vi "ReadBOTUpdates.vi"(0 "reference in":refnum<class "TelegramBOT.lvclass">, 5 "error in (no error)":errorcluster) -> (14 "reference out":refnum<class "TelegramBOT.lvclass">, 16 "result":T1[](array[typedef]), 17 "Connection":bool, 19 "error out":errorcluster)   [LabVIEW 2014, in "TelegramBOT.lvclass"]
uses:
  TelegramBOT.lvclass
  UpdateResultElem.ctl
  QueryStringElem.ctl
  <vilib>/httpClient/LabVIEWHTTPClient.lvlib
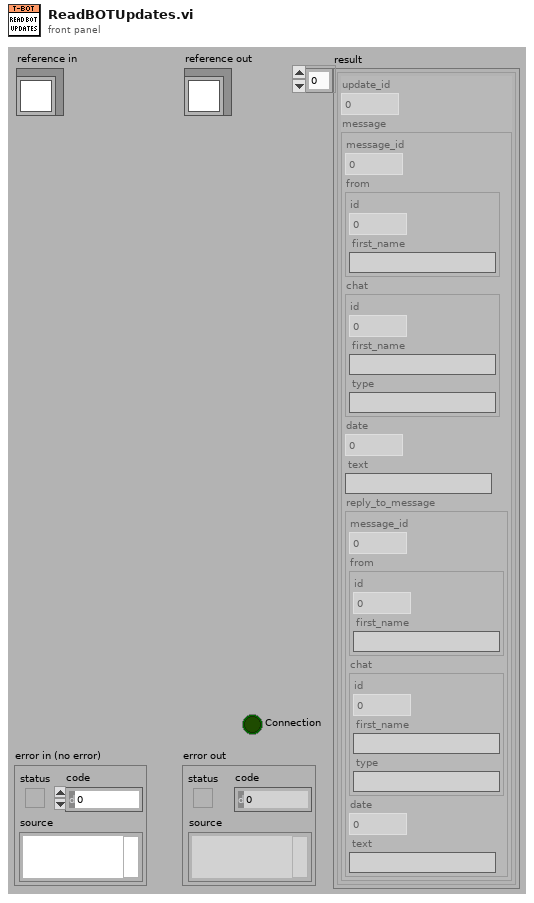
[diagram p1: front panel]
types:
  T1 = typedef "TelegramBOT.lvclass/UpdateResultElem.ctl" = cluster{"update_id":u32, "message":cluster{"message_id":u32, "from":cluster{"id":u64, "first_name":string}, "chat":cluster{"id":i32, "first_name":string, "type":string}, "date":u32, "text":string, "reply_to_message":cluster{"message_id":u32, "from":cluster{"id":u64, "first_name":string}, "chat":cluster{"id":i32, "first_name":string, "type":string}, "date":u32, "text":string}}}
  T2 = typedef "TelegramBOT.lvclass/QueryStringElem.ctl" = cluster{"QueryString":string, "QueryStringValue":string}
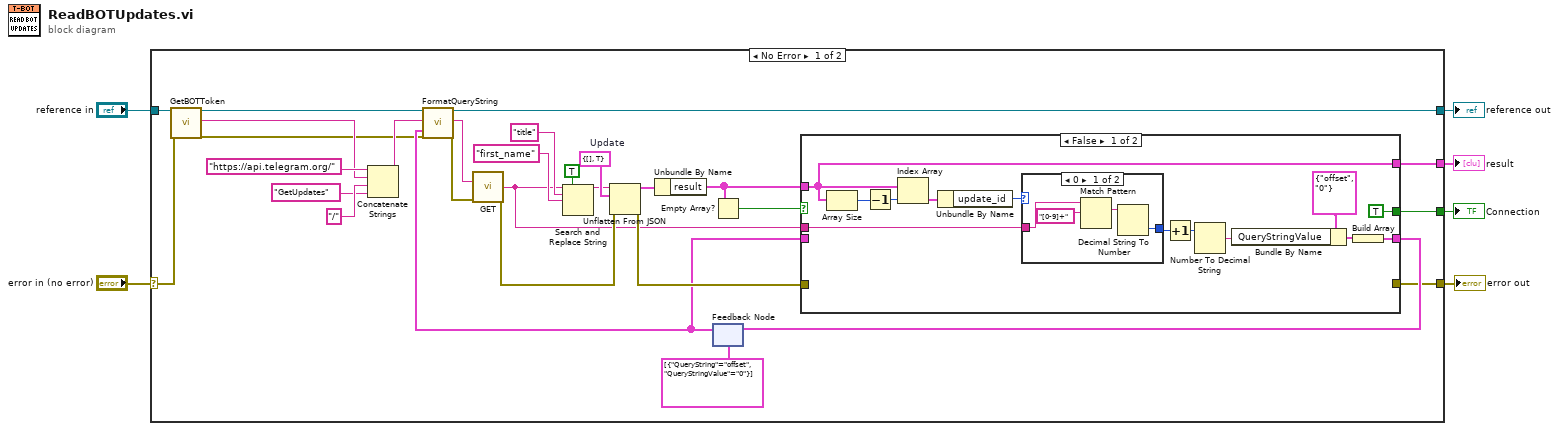
[diagram p0: block diagram]
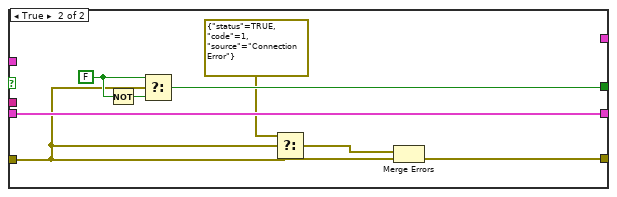
[diagram p3: hidden frame]
diagram:
  n1 = case shown="No Error" "error in (no error)" {
    selector: "error in (no error)" -> [w34 w63]
    tunnel: [w10 w63] -> w5
    tunnel: [w13 w62] -> w3
    tunnel: "reference in" -> [w35 w62]
    tunnel: [w8 _] -> w2
    tunnel: [w7 _] -> w1
    frame No Error {
      w32 = cluster{"result":T1[], "ok":bool} {"result"=[], "ok"=TRUE}  # Update
      n2 = call "GetBOTToken.vi"("reference in"=w35, "error in (no error)"=w34) -> ("reference out"=w14:refnum<class "TelegramBOT.lvclass">, "BOTToken"=w19:string, "error out"=w12:errorcluster)  [unwired: 15 in]
      n3 = Concatenate Strings("https://api.telegram.org/" ("URL"), w19, "/" ("URL"), "GetUpdates" ("URL")) -> (w17:string)
      n4 = feedback #1(T2[] [{"QueryString"="offset", "QueryStringValue"="0"}] ("QueryStringItems")) -> (w15:T2[])
      n5 = call "FormatQueryString.vi"("reference in"=w14, "QueryStringIn"=w17, "QueryStringItems"=w15, "error in (no error)"=w12) -> ("reference out"=w13:refnum<class "TelegramBOT.lvclass">, "QueryStringOut"=w16:string, "error out"=w11:errorcluster)  [unwired: 13 in]
      n6 = call <vilib>:"GET.vi"("url"=w16, "error in (no error)"=w11) -> ("body"=w21:string, "error out"=w27:errorcluster)  [unwired: 10 in, 2 out]
      n7 = Search and Replace String(replace all?=TRUE ("replace all? (F)"), input string=w21, search string="title" ("input string"), replace string="first_name" ("input string")) -> (result string=w28:string)  [unwired: 4 in, 3 out]
      n8 = Unflatten From JSON(JSON string=w28, type and defaults=w32, error in (no error)=w27) -> (value=w24:cluster{"result":T1[], "ok":bool}, error out=w26:errorcluster)  [unwired: 4 in]
      n9 = Unbundle By Name(w24) -> ("result"=w25:T1[])
      n10 = Empty Array?(array=w25) -> (empty?=w23:bool)
      n11 = case shown="False" w23 {
        tunnel: w25 -> [w41 _]
        tunnel: [w45 w61] -> w33
        tunnel: w15 -> [_ w61]
        tunnel: [w41 _] -> w8
        tunnel: w26 -> [_ w56]
        tunnel: [_ w60] -> w10
        tunnel: w21 -> [w42 _]
        tunnel: [TRUE ("status") w57] -> w7
        frame False {
          n12 = Array Size(array=w41) -> (size(s)=w48:i32)
          n13 = Decrement(x=w48) -> (x-1=w47:i32)
          n14 = Index Array(array=w41, index=w47) -> (element=w43:T1)
          n15 = Unbundle By Name(w43) -> ("update_id"=w44:u32)
          n16 = case shown="0" w44 {
            selector: w44 -> [_ w53]
            tunnel: w42 -> [w50 _]
            tunnel: [w49 w53] -> w38
            frame 0 {
              n17 = Match Pattern(string=w50, regular expression="[0-9]+") -> (match substring=w51:string)  [unwired: 1 in, 3 out]
              n18 = Decimal String To Number(string=w51) -> (number=w49:i32)  [unwired: 2 in, 1 out]
            }
            frame Default {
            }
          }
          n19 = Increment(x=w38) -> (x+1=w39:u32)
          n20 = Number To Decimal String(number=w39) -> (decimal integer string=w37:string)  [unwired: 1 in]
          n21 = Bundle By Name(cluster=T2 {"QueryString"="offset", "QueryStringValue"="0"} ("Cluster 2"), "QueryStringValue"=w37) -> (w46:T2)
          n22 = Build Array(w46) -> (w45:T2[])
        }
        frame True {
          w58 = FALSE ("status")
          n23 = Not(x=w58) -> (.not. x?=w59:bool)
          n24 = Select(t=w58, s=w56, f=w59) -> (s? t:f=w57:bool)
          n25 = Select(t=errorcluster {"status"=TRUE, "code"=1, "source"="Connection Error"} ("error in"), s=w56, f=w56) -> (s? t:f=w54:errorcluster)
          n26 = Merge Errors(w54, w56) -> (w60:errorcluster)
        }
      }
      n27 = feedback-in #1(w33) -> ()
    }
    frame Error {
    }
  }
  "error out" <- w5
  "reference out" <- w3
  "result" <- w2
  "Connection" <- w1
